vi "Subscribe Wrapper.vi"(8 "error in (no error)":errorcluster, 10 "key":string="myhome/kitchen/temp", 11 "Session in":u64) -> (0 "error out":errorcluster, 2 "Reader Handle":u64)   [LabVIEW 2021, in "Zenoh.lvclass"]
uses:
  Zenoh.lvclass
  typedef/Zenoh Errors.ctl
  <vilib>/CIF Foundation/CIF Utilities/Errors/Append Error Location.vi
  Zenoh.lvclass/Zenoh.ctl
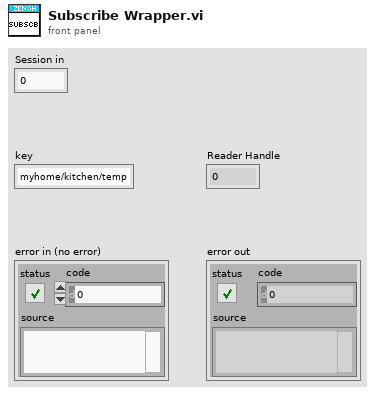
[diagram p1: front panel]
types:
  T1 = typedef "Zenoh.lvclass/Zenoh Errors.ctl" = enum16{"Open Session Error", "Open Subscription Error", "Declare Liveliness"}
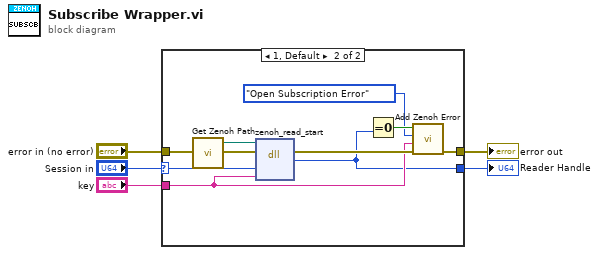
[diagram p0: block diagram]
diagram:
  n1 = case shown="1, Default" "Session in" {
    selector: "Session in" -> [_ w8]
    tunnel: [w6 w15] -> w5
    tunnel: "error in (no error)" -> [w6 w11]
    tunnel: [_ w7] -> w3
    tunnel: "key" -> [_ w9]
    frame 0 {
    }
    frame 1, Default {
      n2 = call "Get Zenoh Path.vi"() -> ("Library Path"=w12:path)  [unwired: 4 in]
      n3 = dll-call lib="C:/Program Files/CIF_Foundation/Libraries/zenoh_lv_wrapper.dll" fn="zenoh_read_start"(path in=w12, error in=w11, "session_prt"=w8, "key"=w9) -> (error out=w10:errorcluster, "ReaderHandle"=w7:u64)  [unwired: 3 in, 1 out]
      n4 = Equal To 0?(x=w7) -> (x = 0?=w14:bool)
      n5 = call "Add Zenoh Error.vi"("error in (no error)"=w10, "String to Append"=w9, "Error"=Zenoh_Errors."Open Subscription Error", "Insert Error"=w14) -> ("error out"=w15:errorcluster)  [unwired: 7 in]
    }
  }
  "error out" <- w5
  "Reader Handle" <- w3
